vi "To Multibyte Char Array.vi"(11 "String":string) -> (3 "Array of Multibyte Chars":string[](array[string]))   [LabVIEW 2017, in "NI_Multibyte Utilities.lvlib"]
doc: "Given a string, return an array of strings where each array element represents one character in the original string. These strings may be multiple bytes long depending upon the character set definition of the current operating system."
uses:
  <vilib>/Utility/Multibyte/NI_Multibyte Utilities.lvlib
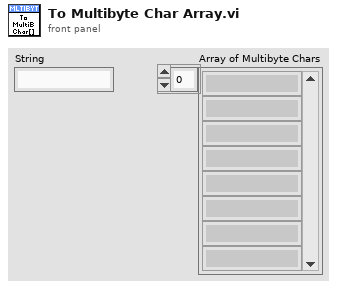
[diagram p1: front panel]
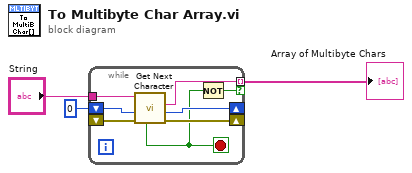
[diagram p0: block diagram]
diagram:
  n1 = while {
    shift-right: [w10] -> _
    shift-left: _ -> [w11]
    shift-right: [w8] -> _
    shift-left: 0 -> [w9]
    tunnel: [w7] -> w2 mode=indexing if=w4
    tunnel: "String" -> [w6]
    stop <- w5 stop-if-true
    n2 = call <vilib>:"Get Next Character.vi"("error in (no error)"=w11, "Offset in"=w9, "String"=w6) -> ("error out"=w10:errorcluster, "Offset out"=w8:i32, "Character"=w7:string, "Past End of String?"=w5:bool)  [unwired: 3 in, 2 out]
    n3 = Not(x=w5) -> (.not. x?=w4:bool)
  }
  "Array of Multibyte Chars" <- w2
